vi "DAQmx.44xx.Get AI Min and Max.vi"(8 "error in (no error)":errorcluster, 9 "AI.channels":tag, 10 "AI.Range":T1) -> (0 "error out":errorcluster, 2 "AI.Max":dbl, 3 "AI.Min":dbl)   [LabVIEW 2019, in "DAQmx.lvclass"]
uses:
  DAQmx.lvclass
  typedefs/DAQ.Config.AI.Range--enum.ctl
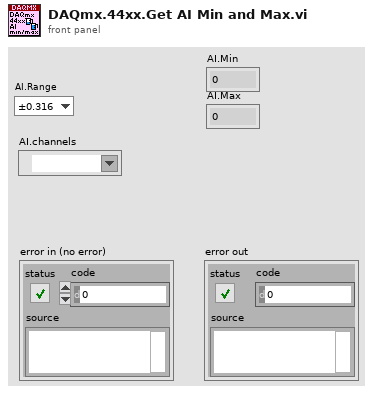
[diagram p1: front panel]
types:
  T1 = typedef "DAQmx.lvclass/DAQ.Config.AI.Range--enum.ctl" = enum16{"±0.316", "±1.00", "±3.16", "±10.0", "±31.6", "±42.4", ""}
  T2 = typedef "DAQmx.lvclass/DAQ.Config.Device Type--enum.ctl" = enum16{"None", "USB-4431", "PXI-446x"}
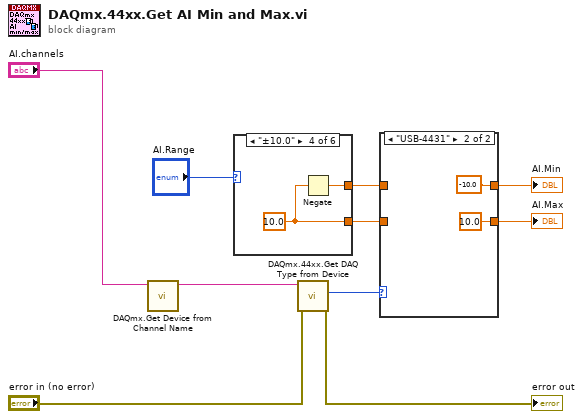
[diagram p0: block diagram]
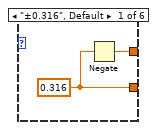
[diagram p2: hidden frame]
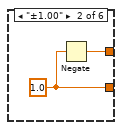
[diagram p3: hidden frame]
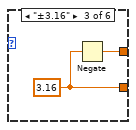
[diagram p4: hidden frame]
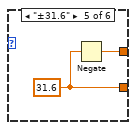
[diagram p5: hidden frame]
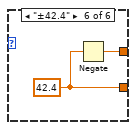
[diagram p6: hidden frame]
diagram:
  n1 = call "DAQmx.Get Device from Channel Name.vi"("Channel"="AI.channels") -> ("Device"=w1:tag)  [unwired: 10 in]
  n2 = case shown="\"±10.0\"" "AI.Range" {
    tunnel: [w11 w13 w15 w17 w19 w21] -> w8
    tunnel: [w12 w14 w16 w18 w20 w22] -> w6
    frame "±0.316", Default {
      w12 = 0.316 ("AI.Min")
      n3 = Negate(x=w12) -> (-x=w11:dbl)
    }
    frame "±1.00" {
      w14 = 1.0 ("AI.Min")
      n4 = Negate(x=w14) -> (-x=w13:dbl)
    }
    frame "±3.16" {
      w16 = 3.16 ("AI.Min")
      n5 = Negate(x=w16) -> (-x=w15:dbl)
    }
    frame "±10.0" {
      w18 = 10.0 ("AI.Min")
      n6 = Negate(x=w18) -> (-x=w17:dbl)
    }
    frame "±31.6" {
      w20 = 31.6 ("AI.Min")
      n7 = Negate(x=w20) -> (-x=w19:dbl)
    }
    frame "±42.4" {
      w22 = 42.4 ("AI.Min")
      n8 = Negate(x=w22) -> (-x=w21:dbl)
    }
  }
  n9 = call "DAQmx.44xx.Get DAQ Type from Device.vi"("error in (no error)"="error in (no error)", "DAQmx Device Name"=w1) -> ("error out"=→"error out":errorcluster, "DAQ Type"=w5:T2)  [unwired: 7 in, 1 out]
  n10 = case shown="\"USB-4431\"" w5 {
    tunnel: [w24 -10.0] -> w9
    tunnel: w8 -> [w24 _]
    tunnel: [w23 10.0 ("AI.Min")] -> w7
    tunnel: w6 -> [w23 _]
    frame Default {
    }
    frame "USB-4431" {
    }
  }
  "AI.Min" <- w9
  "AI.Max" <- w7
